vi "Настройки мишени (Sub VI).vi"(2 "Параметры мишени вх":T1, 5 "error in":errorcluster) -> (16 "Параметры мишени вых":T1, 19 "error out":errorcluster)   [LabVIEW 2013]
doc: "Подпрограмма управления мишенями: создание новой мишени и редактирование существующих"
panel:
  in  "счетчик мишеней":u8
  out "Number of Items":u32
  in  "Удалить мишень":bool
  in  "Отмена":bool
  in  "Y0":u16
  in  "Х0":u16
  in  "Добавить мишень":bool
  in  "Ширина, мм":u8
  in  "Длина, мм":u8
  in  "Мишень":u16(ring) items=["1"]
  in  "Сохранить настройки":bool
  # "Настройки"
  # "Положение"
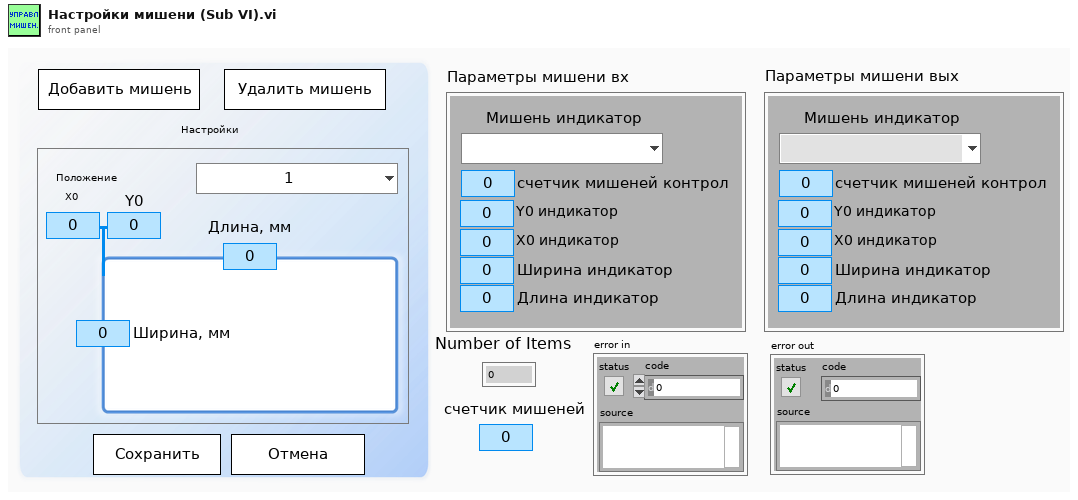
[diagram p1: front panel]
types:
  T1 = cluster{"Мишень индикатор":u16, "счетчик мишеней контрол":u8, "Ширина индикатор":u8, "Длина индикатор":u8, "Y0 индикатор":u16, "X0 индикатор":u16}
  T2 = typedef "LVStringsAndValuesArrayTypeDef_U16.ctl" = cluster{"String":string, "Value":u16}[]
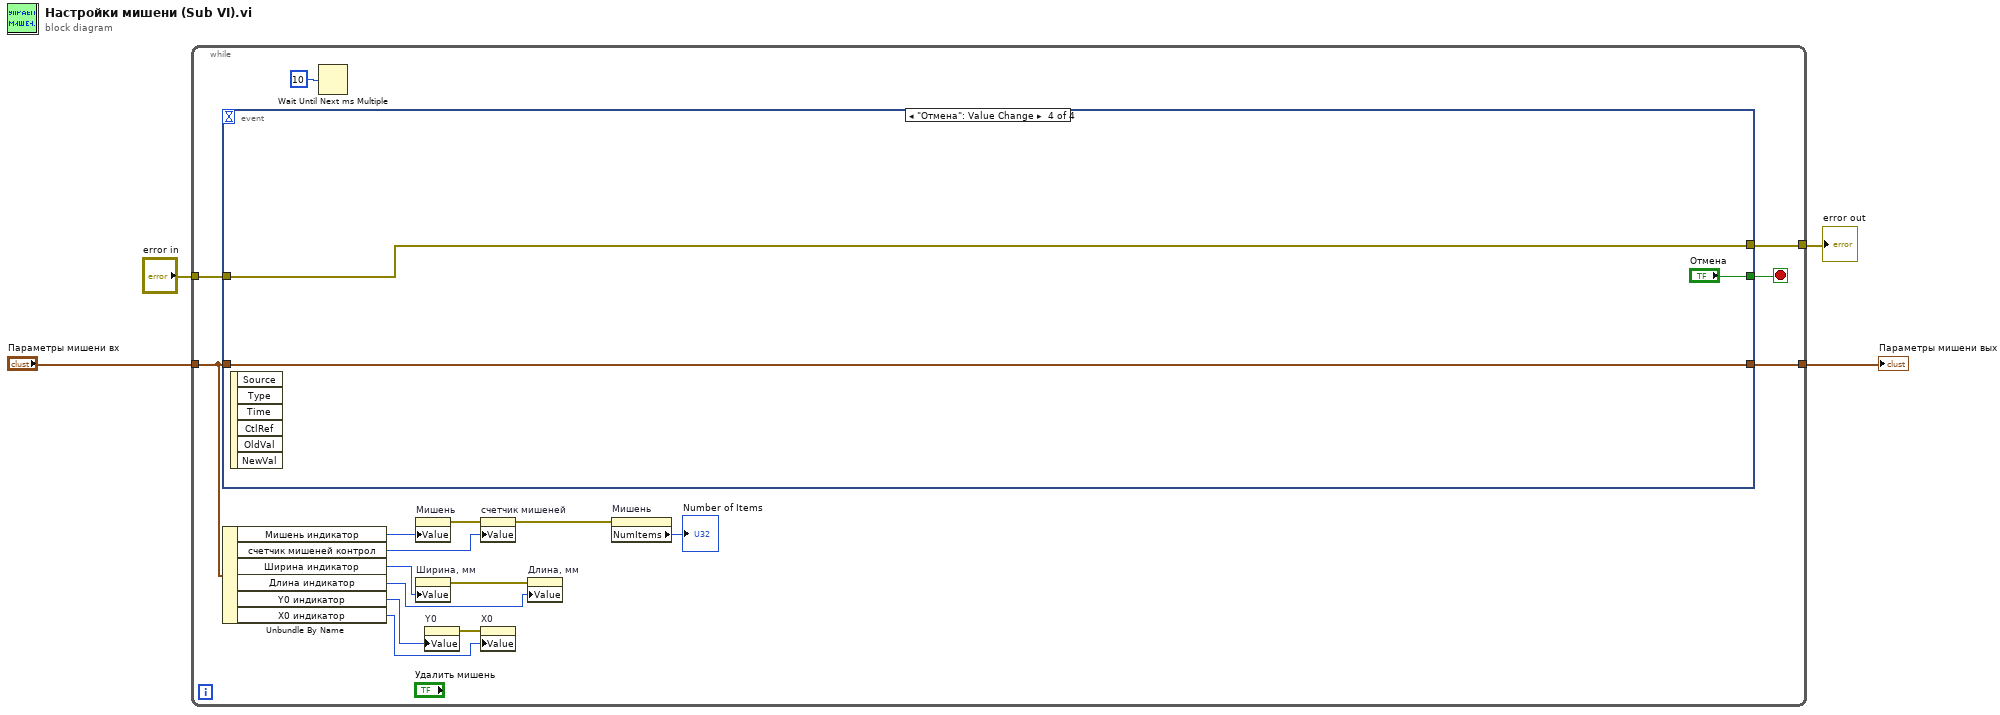
[diagram p0: block diagram]
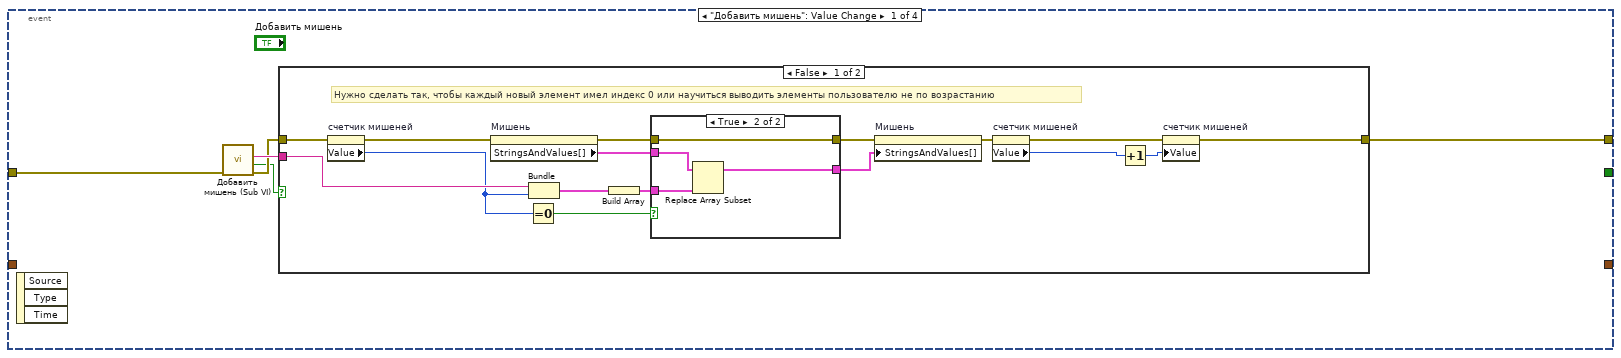
[diagram p2: hidden frame]
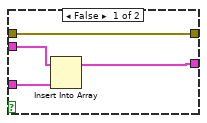
[diagram p3: hidden frame]
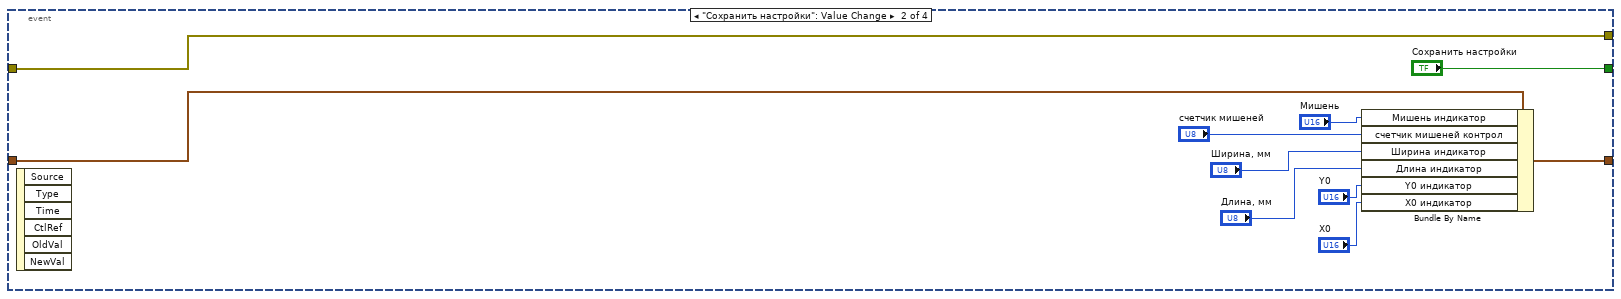
[diagram p5: hidden frame]
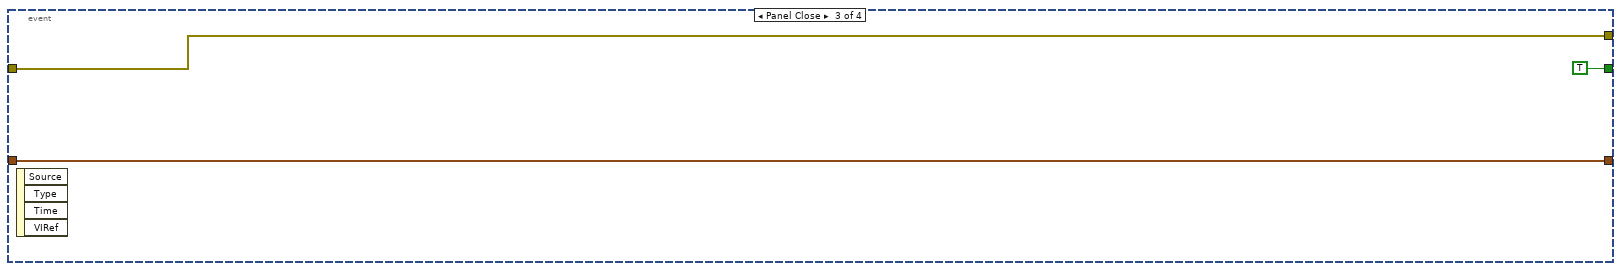
[diagram p6: hidden frame]
diagram:
  n1 = while {
    tunnel: [w8] -> w4
    tunnel: [w7] -> w3
    tunnel: "Параметры мишени вх" -> [w6]
    tunnel: "error in" -> [w5]
    stop <- w10 stop-if-true
    n2 = event shown="[3] \"Отмена\": Value Change" {
      selector: _ -> [_ _ _ _]
      dyn-events: _ -> [_ _ _ _]
      timeout: _ -> [_ _ _ _]
      tunnel: w6 -> [_ w55 w64 w67]
      tunnel: [_ w54 w64 w67] -> w7
      tunnel: [w23 w53 w63 w66] -> w8
      tunnel: w5 -> [w22 w53 w63 w66]
      tunnel: [_ "Сохранить настройки" TRUE ("Сохранить настройки") "Отмена"] -> w10
      event "Добавить мишень": Value Change {
        n3 = event-data() -> ()  [unwired: 1 in, 3 out]
        n4 = call "Добавить мишень (Sub VI).vi"("error in"=w22) -> ("error out"=w25:errorcluster, "отменен?"=w24:bool, "Название мишени"=w26:string)  [unwired: 8 in]
        n5 = case shown="False" w24 {
          tunnel: w26 -> [w42 _]
          tunnel: w25 -> [w39 w51]
          tunnel: [w27 w51] -> w23
          frame False {
            # "Нужно сделать так, чтобы каждый новый элемент имел индекс 0 или научиться выводить элементы пользователю не по возрастанию"
            n6 = property on="счетчик мишеней" class="DigNum (strict)"(error in=w39) -> (error out=w40:errorcluster, "Value"=w37:u8)  [unwired: 1 in, 1 out]
            n7 = property on="Мишень" class="Ring (strict)"(error in=w40) -> (error out=w36:errorcluster, "StringsAndValues[]"=w28:T2)  [unwired: 1 in, 1 out]
            n8 = Equal To 0?(x=w37) -> (x = 0?=w38:bool)
            n9 = Bundle("Название мишени"=w42, "Value"=w37) -> (w41:cluster{"Название мишени":string, "Value":u8})  [unwired: 1 in]
            n10 = Build Array(w41) -> (w35:cluster{"Название мишени":string, "Value":u8}[])
            n11 = case shown="True" w38 {
              tunnel: w28 -> [w43 w50]
              tunnel: [w46 w49] -> w29
              tunnel: w35 -> [w45 w48]
              tunnel: [w44 w47] -> w30
              tunnel: w36 -> [w44 w47]
              frame False {
                n12 = Insert Into Array "Insert Into Array"(array=w43, new element=w45) -> (w46:T2)  [unwired: 1 in]
              }
              frame True {
                n13 = Replace Array Subset "Replace Array Subset"(array=w50, new element=w48) -> (w49:T2)  [unwired: 1 in]
              }
            }
            n14 = property on="Мишень" class="Ring (strict)"(error in=w30, "StringsAndValues[]"=w29) -> (error out=w31:errorcluster)  [unwired: 1 in, 1 out]
            n15 = property on="счетчик мишеней" class="DigNum (strict)"(error in=w31) -> (error out=w32:errorcluster, "Value"=w33:u8)  [unwired: 1 in, 1 out]
            n16 = Increment(x=w33) -> (x+1=w34:u8)
            n17 = property on="счетчик мишеней" class="DigNum (strict)"(error in=w32, "Value"=w34) -> (error out=w27:errorcluster)  [unwired: 1 in, 1 out]
          }
          frame True {
          }
        }
      }
      event "Сохранить настройки": Value Change {
        n18 = event-data() -> ()  [unwired: 1 in, 6 out]
        n19 = Bundle By Name(cluster=w55, "Мишень индикатор"="Мишень", "счетчик мишеней контрол"="счетчик мишеней", "Ширина индикатор"="Ширина, мм", "Длина индикатор"="Длина, мм", "Y0 индикатор"="Y0", "X0 индикатор"="Х0") -> (w54:T1)
      }
      event Panel Close {
        n20 = event-data() -> ()  [unwired: 1 in, 4 out]
      }
      event "Отмена": Value Change {
        n21 = event-data() -> ()  [unwired: 1 in, 6 out]
      }
    }
    n22 = Unbundle By Name(w6) -> ("Мишень индикатор"=w20:u16, "счетчик мишеней контрол"=w19:u8, "Ширина индикатор"=w18:u8, "Длина индикатор"=w17:u8, "Y0 индикатор"=w16:u16, "X0 индикатор"=w15:u16)
    n23 = Wait Until Next ms Multiple(millisecond multiple=u32 10) -> ()  [unwired: 1 out]
    n24 = property on="Мишень" class="Ring (strict)"("Value"=w20) -> (error out=w14:errorcluster)  [unwired: 2 in, 1 out]
    n25 = property on="Ширина, мм" class="DigNum (strict)"("Value"=w18) -> (error out=w13:errorcluster)  [unwired: 2 in, 1 out]
    n26 = property on="Y0" class="DigNum (strict)"("Value"=w16) -> (error out=w12:errorcluster)  [unwired: 2 in, 1 out]
    n27 = property on="счетчик мишеней" class="DigNum (strict)"(error in=w14, "Value"=w19) -> (error out=w11:errorcluster)  [unwired: 1 in, 1 out]
    n28 = property on="Х0" class="DigNum (strict)"(error in=w12, "Value"=w15) -> ()  [unwired: 1 in, 2 out]
    n29 = property on="Длина, мм" class="DigNum (strict)"(error in=w13, "Value"=w17) -> ()  [unwired: 1 in, 2 out]
    n30 = property on="Мишень" class="Ring (strict)"(error in=w11) -> ("NumItems"=→"Number of Items":u32)  [unwired: 1 in, 2 out]
  }
  "error out" <- w4
  "Параметры мишени вых" <- w3
